vi "Kelvinox_Open_Queue.vi"(8 "error in (no error)":errorcluster) -> (0 "error out":errorcluster, 2 "queue out":refnum<queue>)   [LabVIEW 2019]
uses:
  Kelvinox/Kelvinox_Control.ctl
  Global/Global Variables/Queues_global.vi
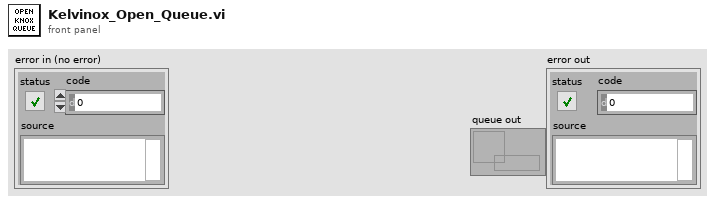
[diagram p1: front panel]
types:
  T1 = typedef "Kelvinox_Control.ctl" = cluster{"T-Setpoint-Manual":dbl, "Rate (K/min)":dbl, "Change T Control Status":bool, "Emergency Stop":bool, "Set Setpoint":bool}
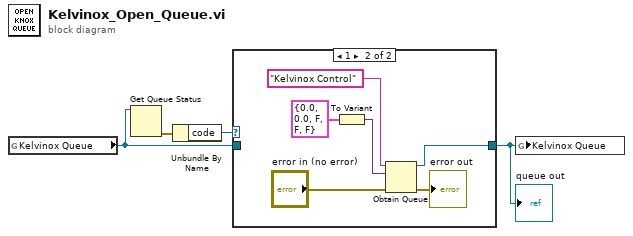
[diagram p0: block diagram]
diagram:
  n1 = global read "Queues_global.vi" "Kelvinox Queue"() -> (w2:refnum<queue>)
  n2 = Get Queue Status(queue=w2) -> (error out=w4:errorcluster)  [unwired: 2 in, 7 out]
  n3 = Unbundle By Name(w4) -> ("code"=w3:i32)
  n4 = case shown="1" w3 {
    tunnel: [w5 w7] -> w1
    tunnel: w2 -> [w5 _]
    frame 0, Default {
    }
    frame 1 {
      n5 = To Variant(anything=T1 {"T-Setpoint-Manual"=0.0, "Rate (K/min)"=0.0, "Change T Control Status"=FALSE, "Emergency Stop"=FALSE, "Set Setpoint"=FALSE} ("Kelvinox-Cluster")) -> (Variant=w10:variant)
      n6 = Obtain Queue(name (unnamed)="Kelvinox Control", element data type=w10, error in (no error)="error in (no error)") -> (queue out=w7:refnum<queue>, error out=→"error out":errorcluster)  [unwired: 2 in, 1 out]
    }
  }
  "queue out" <- w1
  n7 = global write "Queues_global.vi" "Kelvinox Queue"(w1) -> ()
